vi "Настройки мишени (Sub VI).vi"(2 "Параметры мишеней вх":T1, 5 "error in":errorcluster) -> (11 "Параметры мишеней вых":T1, 19 "error out":errorcluster)   [LabVIEW 2015]
doc: "Подпрограмма управления мишенями: создание новой мишени и редактирование существующих"
panel:
  in  "Настройки мишени:":string
  in  "Ширина, мм":u16 max=60
  in  "Длина, мм":u16 max=100
  in  "Шаг перехода по вертикали":dbl min=0.0 max=60.0 format="%.1f"
  in  "Шаг перехода по горизонтали":dbl min=0.0 max=100.0 format="%.1f"
  in  "Выстрелов до перехода":u16
  in  "Отмена":bool
  in  "Y0":u16 max=60
  in  "Х0":u16 max=100
  in  "Сохранить настройки":bool
  # "Положение:"
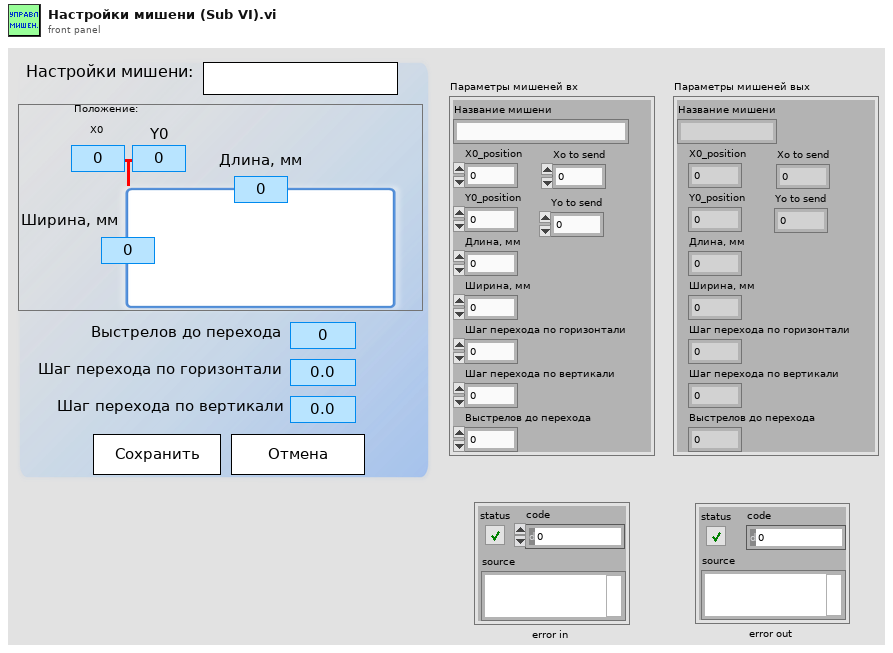
[diagram p1: front panel]
types:
  T1 = cluster{"Название мишени":string, "Х0_position":u16, "Y0_position":u16, "Длина, мм":u16, "Ширина, мм":u16, "Шаг перехода по горизонтали":dbl, "Шаг перехода по вертикали":dbl, "Выстрелов до перехода":u16, "Xo to send ":u16, "Yo to send":u16}
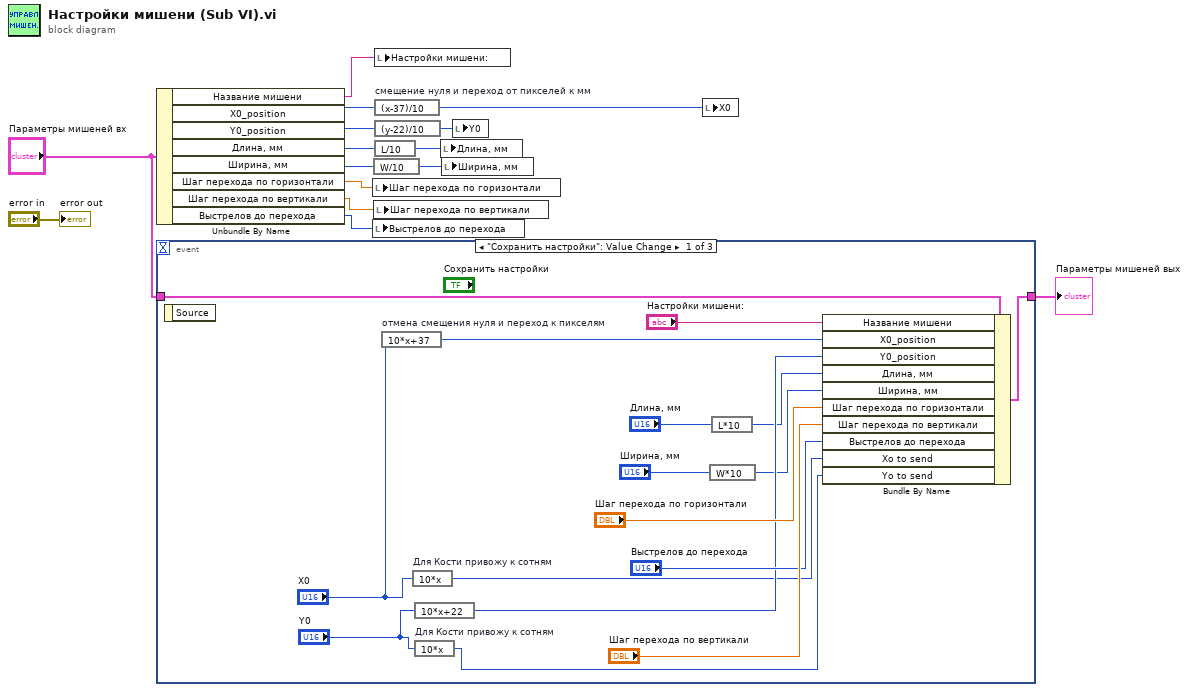
[diagram p0: block diagram]
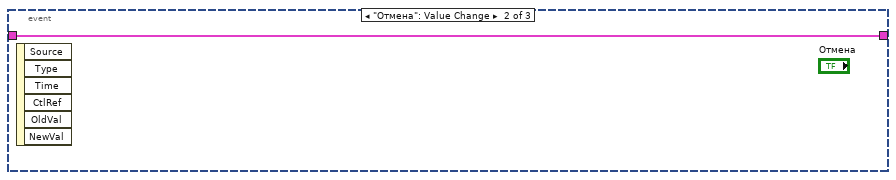
[diagram p2: hidden frame]
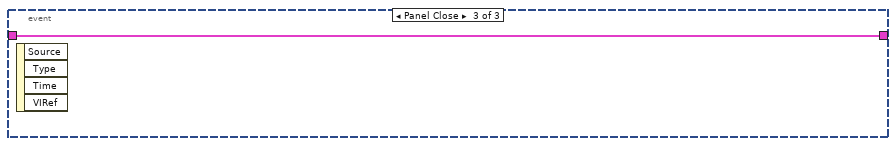
[diagram p3: hidden frame]
diagram:
  n1 = Unbundle By Name("Параметры мишеней вх") -> ("Название мишени"=w12:string, "Х0_position"=w8:u16, "Y0_position"=w7:u16, "Длина, мм"=w4:u16, "Ширина, мм"=w2:u16, "Шаг перехода по горизонтали"=w11:dbl, "Шаг перехода по вертикали"=w10:dbl, "Выстрелов до перехода"=w9:u16)
  n2 = event shown="[0] \"Сохранить настройки\": Value Change" {
    selector: _ -> [_ _ _]
    dyn-events: _ -> [_ _ _]
    timeout: _ -> [_ _ _]
    tunnel: [w31 w32 w33] -> w14
    tunnel: "Параметры мишеней вх" -> [w30 w32 w33]
    event "Сохранить настройки": Value Change {
      n3 = event-data() -> ()  [unwired: 1 in, 1 out]
      n4 = expression code="10*x+37" "отмена смещения нуля и переход к пикселям"("Х0") -> (w25:u16)
      n5 = expression code="10*x" "Для Кости привожу к сотням"("Х0") -> (w18:u16)
      n6 = expression code="10*x+22"("Y0") -> (w24:u16)
      n7 = expression code="10*x" "Для Кости привожу к сотням"("Y0") -> (w16:u16)
      n8 = expression code="W*10"("Ширина, мм") -> (w21:u16)
      n9 = expression code="L*10"("Длина, мм") -> (w23:u16)
      n10 = Bundle By Name(cluster=w30, "Название мишени"="Настройки мишени:", "Х0_position"=w25, "Y0_position"=w24, "Длина, мм"=w23, "Ширина, мм"=w21, "Шаг перехода по горизонтали"="Шаг перехода по горизонтали", "Шаг перехода по вертикали"="Шаг перехода по вертикали", "Выстрелов до перехода"="Выстрелов до перехода", "Xo to send"=w18, "Yo to send"=w16) -> (w31:T1)
    }
    event "Отмена": Value Change {
      n11 = event-data() -> ()  [unwired: 1 in, 6 out]
    }
    event Panel Close {
      n12 = event-data() -> ()  [unwired: 1 in, 4 out]
    }
  }
  "Параметры мишеней вых" <- w14
  n13 = local write "Шаг перехода по горизонтали"(w11) -> ()
  n14 = local write "Выстрелов до перехода"(w9) -> ()
  n15 = expression code="W/10"(w2) -> (w1:u16)
  n16 = local write "Шаг перехода по вертикали"(w10) -> ()
  n17 = local write "Настройки мишени:"(w12) -> ()
  n18 = expression code="(x-37)/10" "смещение нуля и переход от пикселей к мм"(w8) -> (w6:u16)
  n19 = expression code="(y-22)/10"(w7) -> (w5:u16)
  n20 = expression code="L/10"(w4) -> (w3:u16)
  n21 = local write "Длина, мм"(w3) -> ()
  n22 = local write "Ширина, мм"(w1) -> ()
  n23 = local write "Y0"(w5) -> ()
  n24 = local write "Х0"(w6) -> ()
  "error out" <- "error in"
